vi "iscan.vi"(0 "IP adress":string="192.109.209.229", 1 "stop":bool, 2 "Channel":u8(ring)=12 items=["1", "2", "3", "4", "5", "6", "7", "8", "9", "10", "11", "12", "13", "14", "15", "16"], 3 "ISCAN Parameters":T1={"vs_initial "=TRUE, "Current_step"=0.0, "Scans"=[{" vs_initial"=FALSE, "Current_step"=0.001, "Scan_Rate"=1.0}, {" vs_initial"=FALSE, "Current_step"=-0.001, "Scan_Rate"=1.0}, {" vs_initial"=FALSE, "Current_step"=0.0, "Scan_Rate"=1.0}], "Scan_number"=2, "N_Cycles"=1, "Record_every_dI"=1e-05, "Begin_measuring_E"=0.5, "End_measuring_I"=0.75, "I_Range"=7, "E_Range"=2, "Bandwidth"=5, "em"=1, "ce"=0, "tb"=5e-05} {"tb" min=5e-05 max=1 format="%^_3e"; "ce" items=["Standard", "CE to ground"]; "End_measuring_I" min=0 max=1 format="%.2f"; "Begin_measuring_E" min=0 max=1 format="%.2f"; "Current_step" min=-150 max=150 format="%^_3e"; "N_Cycles" min=0 max=1000000; "Scan_number" min=0 max=98; "Scans"."Scan_Rate" min=0.01 max=1000 format="%^_3e"; "Scans"."Current_step" min=-150 max=150 format="%^_3e"; "E_Range" items=["±2.5V", "±5V", "±10V", "Auto"]; "Bandwidth" items=["1"=1, "2"=2, "3"=3, "4"=4, "5"=5, "6"=6, "7"=7, "8"=8, "9"=9]; "Record_every_dI" format="%^_3e"; "I_Range" items=["1pA", "1nA", "10nA", "100nA", "1µA", "10µA", "100µA", "1mA", "10mA", "100mA", "1A", "Booster"]}, 4 "Exit":bool, 5 "Start":bool, 6 "Draw":enum16{"I(Ewe)", "Ewe(t)", "I(t)"}(ring)=enum."I(t)") -> (7 "XY Graph":cluster{"Data 101":sgl[], "Data 101":sgl[]}(graph), 8 "Number of points":i32=105)   [LabVIEW 2012]
doc: "The Current scan technique (Galvanodynamic Technique) technique allows the user to perform galvanodynamic periods with different scan rates.\nIn general, in this VI, the first thing to do is to start by establishing the connection with the instrument defined by its IP adress, then load the firmware in the channel selected, get the information on the plugged channels, load protocol on a channel, start/stop the protocol, retreive data and draw the graph."
uses:
  base_xml.llb/Type Descriptor Enumeration__ogtk.ctl
panel:
  out "Device Code":i32
  out "Exit 2":bool=TRUE
  out "Data 125":sgl[][](array[numeric])=[[0.003, 0.0019739384, 6.01559e-07, 0.002076381], [0.105000004, 0.012167796, 2.1901733e-06, 0.0117511805], [0.20700002, 0.022361653, 3.975648e-06, 0.021977918], [0.30900002, 0.03255551, 5.772186e-06, 0.032090176], [0.411, 0.042749364, 7.5965745e-06, 0.042278755], [0.513, 0.052943222, 9.43279e-06, 0.052619968], [0.615, 0.06313708, 1.1011484e-05, 0.06277039], [0.717, 0.07333094, 1.3262951e-05, 0.07292081], [0.81900007, 0.08352479, 1.5135982e-05, 0.082956746], [0.92, 0.09371865, 1.6970866e-05, 0.09329796], [1.146, 0.08352479, 1.50444275e-05, 0.083796255], [1.248, 0.07333094, 1.3190472e-05, 0.07337872], [1.35, 0.06313708, 1.1359403e-05, 0.06338094], [1.4510001, 0.052943222, 9.505447e-06, 0.053039722], [1.5530001, 0.042749364, 7.704897e-06, 0.042965624], [1.6550001, 0.03255551, 5.7821057e-06, 0.03273889], [1.7570001, 0.022361653, 3.9939605e-06, 0.02243583], [1.8590001, 0.012167796, 2.2004742e-06, 0.012209094], [1.9610001, 0.0019739384, 3.9210917e-07, 0.0019060377], [2.0630002, -0.008219917, -1.42999e-06, -0.007939104], [2.1650002, -0.018413773, -3.2925293e-06, -0.01812768], [2.2670002, -0.02860763, -5.1661327e-06, -0.028087301], [2.3690002, -0.038801484, -7.0229494e-06, -0.038695633], [2.4710002, -0.048995342, -8.872135e-06, -0.048960526], [2.5730002, -0.059189197, -1.0682789e-05, -0.059149105], [2.6750002, -0.069383055, -1.2368184e-05, -0.06929952], [2.7770002, -0.07957691, -1.4145845e-05, -0.079564415], [2.8790002, -0.089770764, -1.595784e-05, -0.08963852], [2.9810002, -0.09996462, -1.7746945e-05, -0.09997973], [3.0830002, -0.11015848, -1.9597086e-05, -0.11005383], [3.1840003, -0.120352335, -2.1420525e-05, -0.1202424], [3.2860003, -0.13054618, -2.3339331e-05, -0.13024017], [3.3880002, -0.14074004, -2.5181842e-05, -0.14054324], [3.4900002, -0.1509339, -2.7039614e-05, -0.15061733], [3.5920002, -0.16112776, -2.8866867e-05, -0.16069143], [3.6940002, -0.17132162, -3.0690302e-05, -0.17118528], [3.7960002, -0.18151547, -3.246415e-05, -0.18129754], [3.8980002, -0.19170932, -3.425326e-05, -0.19167691], [4.1660004, -0.18151547, -3.2410746e-05, -0.1819081], [4.268, -0.17132162, -3.064834e-05, -0.17160504], [4.3700004, -0.16112776, -2.8840164e-05, -0.1615691], [4.472, -0.1509339, -2.6993837e-05, -0.15141869], [4.5740004, -0.14074004, -2.5170399e-05, -0.14126827], [4.676, -0.13054618, -2.3297369e-05, -0.13085073], [4.7780004, -0.120352335, -2.1454858e-05, -0.120471366], [4.88, -0.11015848, -1.9608531e-05, -0.11066438], [4.9820004, -0.09996462, -1.7731685e-05, -0.100361325], [5.084, -0.089770764, -1.5908246e-05, -0.09028722], [5.1860003, -0.07957691, -1.4138216e-05, -0.07979337], [5.288, -0.069383055, -1.23643695e-05, -0.06975743], [5.3900003, -0.059189197, -1.0510413e-05, -0.059530698], [5.491, -0.048995342, -8.728937e-06, -0.049342122], [5.5930004, -0.038801484, -6.897869e-06, -0.039191704], [5.695, -0.02860763, -5.1615543e-06, -0.029041288], [5.7970004, -0.018413773, -3.292148e-06, -0.018547434], [5.899, -0.008219917, -1.4265564e-06, -0.008549656], [6.0010004, 0.0019739384, 4.397981e-07, 0.0014481241], [6.103, 0.012167796, 2.245111e-06, 0.011636702], [6.2050004, 0.022361653, 4.0595805e-06, 0.021939758], [6.307, 0.03255551, 5.846962e-06, 0.032090176], [6.4090004, 0.042749364, 7.638159e-06, 0.04212612], [6.511, 0.052943222, 9.431646e-06, 0.05246733], [6.6130004, 0.06313708, 1.1045057e-05, 0.062579595], [6.715, 0.07333094, 1.3209546e-05, 0.07276817], [6.8170004, 0.08352479, 1.5067316e-05, 0.08303307], [6.919, 0.09371865, 1.690983e-05, 0.09318349], [7.1440005, 0.08352479, 1.5128351e-05, 0.08364362], [7.2460003, 0.07333094, 1.3301099e-05, 0.0733024], [7.3480005, 0.06313708, 1.1408995e-05, 0.06338094], [7.4490004, 0.052943222, 9.520706e-06, 0.053039726], [7.5510006, 0.042749364, 7.704897e-06, 0.042316914], [7.6530004, 0.03255551, 5.7290754e-06, 0.032624412], [7.7550006, 0.022361653, 3.9203287e-06, 0.02262663], [7.8570004, 0.012167796, 2.1073854e-06, 0.012056456], [7.9590006, 0.0019739384, 3.3221184e-07, 0.0022876323], [8.061001, -0.008219917, -1.4410538e-06, -0.007900944], [8.163, -0.018413773, -3.2478924e-06, -0.017975042], [8.265, -0.02860763, -5.089448e-06, -0.028316258], [8.367001, -0.038801484, -6.929479e-06, -0.038504835], [8.469001, -0.048995342, -8.814146e-06, -0.04869341], [8.571, -0.059189197, -1.0662569e-05, -0.059263583], [8.673, -0.069383055, -1.2417775e-05, -0.06933768], [8.775001, -0.07957691, -1.42297695e-05, -0.079144664], [8.877001, -0.089770764, -1.6053207e-05, -0.0893714], [8.979, -0.09996462, -1.7861388e-05, -0.09982709], [9.081, -0.11015848, -1.9642863e-05, -0.10990119], [9.182, -0.120352335, -2.1462487e-05, -0.12020425], [9.284, -0.13054618, -2.3247778e-05, -0.13043097], [9.386001, -0.14074004, -2.5071215e-05, -0.14046691], [9.488001, -0.1509339, -2.6944244e-05, -0.15084629], [9.59, -0.16112776, -2.8832534e-05, -0.16084407], [9.692, -0.17132162, -3.0682673e-05, -0.17129977], [9.794001, -0.18151547, -3.2525186e-05, -0.18110675], [9.896001, -0.19170932, -3.435244e-05, -0.19156244], [10.1640005, -0.18151547, -3.2357337e-05, -0.18206073], [10.266001, -0.17132162, -3.0552972e-05, -0.1716432], [10.368, -0.16112776, -2.8763869e-05, -0.16137831], [10.47, -0.1509339, -2.6936617e-05, -0.15138052], [10.5720005, -0.14074004, -2.5143696e-05, -0.14138275], [10.674001, -0.13054618, -2.3377479e-05, -0.1306981], [10.776001, -0.120352335, -2.1515893e-05, -0.12066216], [10.878, -0.11015848, -1.9719157e-05, -0.11047359], [10.9800005, -0.09996462, -1.780798e-05, -0.100513965], [11.082001, -0.089770764, -1.5946394e-05, -0.09021091], [11.184001, -0.07957691, -1.4088625e-05, -0.079869695]] format="%.2f"
  # "Instructions:\nBefore running the VI you must type a valid IP adress that corresponds to the instrument.Then press the Run button to execute this VI.\nWhile this VI is running, choose the available channel, enter the ISCAN parameters or keep the default values, then press the button start to begin the experience.\nChoose the waveform to draw (Ewe(t) or I(t) or I(Ewe) or Ec(t). You can stop the measure if you press the stop button and exit the execution if you press the exit button."
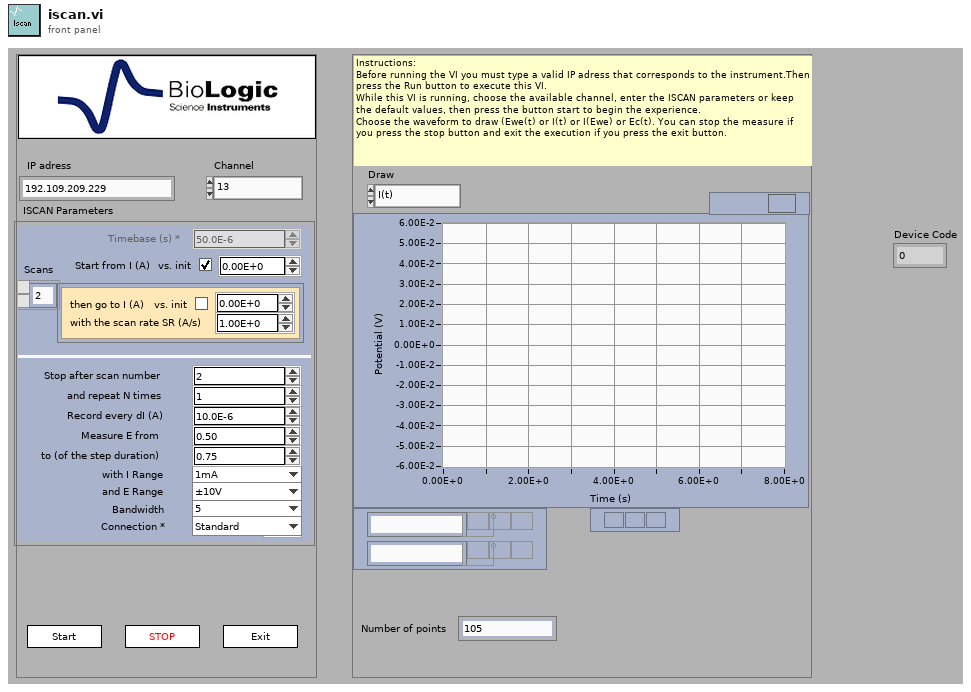
[diagram p1: front panel]
types:
  T1 = cluster{"vs_initial ":bool, "Current_step":sgl, "Scans":cluster{" vs_initial":bool, "Current_step":sgl, "Scan_Rate":sgl}[], "Scan_number":i32, "N_Cycles":i32, "Record_every_dI":sgl, "Begin_measuring_E":sgl, "End_measuring_I":sgl, "I_Range":u16, "E_Range":u16, "Bandwidth":u16, "em":u16, "ce":u16, "tb":sgl}
  T2 = typedef "Type Descriptor Enumeration__ogtk.ctl" = enum8{"<Null>", "I8", "I16", "I32", "I64", "U8", "U16", "U32", "U64", "SGL", "DBL", "EXT", "CSG", "CDB", "CXT", "0x0F", "0x10", "0x11", "0x12", "0x13", "0x14", "Enum U8", "Enum U16", "Enum U32", "Enum U64", "SGL PQ", "DBL PQ", "EXT PQ", "CSG PQ", "CDB PQ", "CXT PQ", "0x1F", "0x20", "Boolean", "0x22", "0x23", "0x24", "0x25", "0x26", "0x27", "0x28", "0x29", "0x2A", "0x2B", "0x2C", "0x2D", "0x2E", "0x2F", "String", "0x31", "Path", "Pict", "0x34", "0x35", "0x36", "DAQ", "0x38", "0x39", "0x3A", "0x3B", "0x3C", "0x3D", "0x3E", "0x3F", "Array", "0x41", "0x42", "0x43", "0x44", "0x45", "0x46", "0x47", "0x48", "0x49", "0x4A", "0x4B", "0x4C", "0x4D", "0x4E", "0x4F", "Cluster", "0x51", "0x52", "Variant", "Waveform", "0x55", "0x56", "0x57", "0x58", "0x59", "0x5A", "0x5B", "0x5C", "0x5D", "0x5E", "0x5F", "0x60", "0x61", "0x62", "0x63", "0x64", "0x65", "0x66", "0x67", "0x68", "0x69", "0x6A", "0x6B", "0x6C", "0x6D", "0x6E", "0x6F", "Refnum"}
  T3 = cluster{"Data Type":T2, "Format String":string}[]
  T4 = cluster{"Channel":i32, "BoardVersion":i32, "BoardSerialCode":i32, "FirmwareCode":i32, "FirmwareVersion":i32, "XilinxVersion":i32, "AmpCode":i32, "NbAmp":i32, "LcBoard":i32, "Zboard":i32, "MuxBoard":i32, "GPRAboard":i32, "MemSize":i32, "MemFilled":i32, "state":i32, "MaxIRange":i32, "MinIRange":i32, "MaxBandwidth":i32, "NbOfTechniques":i32}
  T5 = cluster{" vs_initial":bool, "Current_step":sgl, "Scan_Rate":sgl}[]
  T6 = cluster{" vs_initial":bool, "Current_step":sgl, "Scan_Rate":sgl}
  T7 = cluster{"Label":string, "type":i32, "valeur":u32, "index":i32}[]
  T8 = cluster{"IRQskipped":i32, "NbRaws":i32, "NbCols":i32, "Technique Index":i32, "TechniqueID":i32, "PrcessIndex":i32, "loop":i32, "StartTime":dbl, "MuxPad":i32}
  T9 = cluster{"State":i32, "MemFilled":i32, "TimeBase":sgl, " Ewe":sgl, " EweRangeMin":sgl, " EweRangeMax":sgl, "Ece":sgl, "EceRangeMin":sgl, "EceRangeMax":sgl, "Eoverflow":i32, "I":sgl, "IRange":i32, "Ioverflow":i32, "ElapsedTime":sgl, "Freq":sgl, "Rcomp":sgl, "Saturation":sgl, "OptErr":i32, "OptPos":i32}
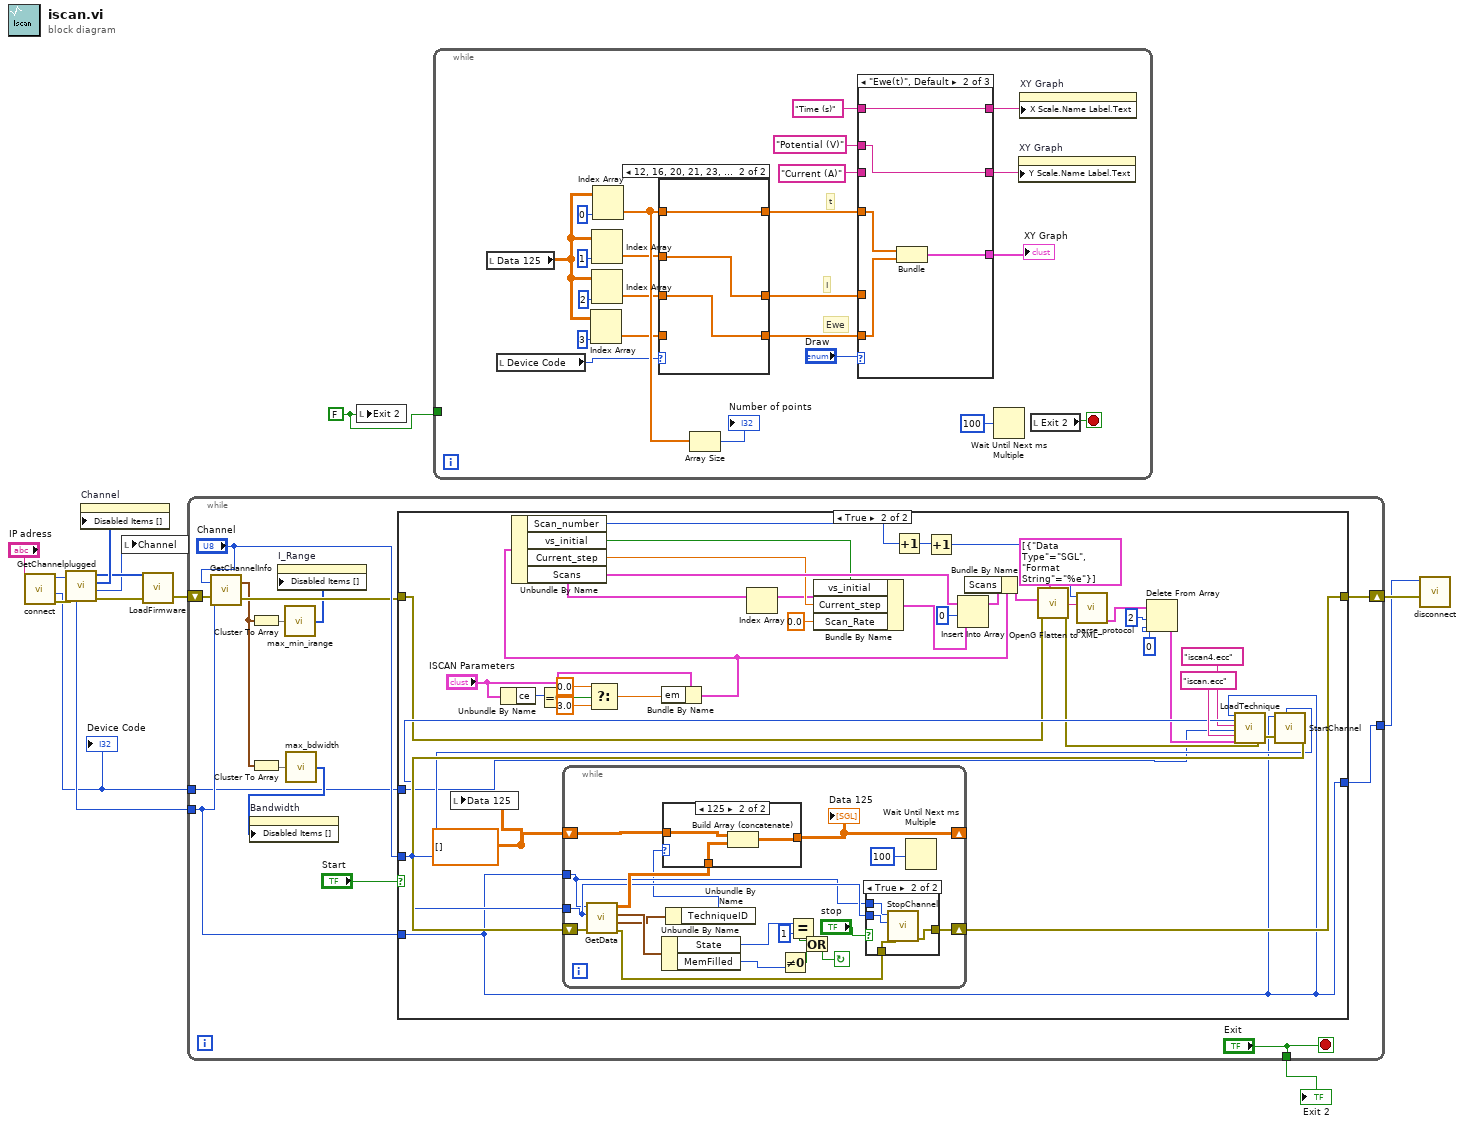
[diagram p0: block diagram]
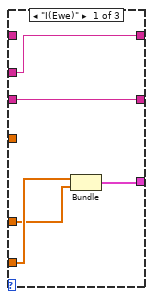
[diagram p3: hidden frame]
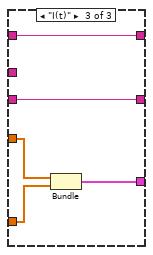
[diagram p4: hidden frame]
diagram:
  w12 = FALSE ("Exit 2")
  n1 = call "connect.vi"("IP"="IP adress") -> ("error out"=w10:errorcluster, "Device Code"=w1:i32, "ID"=w3:i32)  [unwired: 7 in, 1 out]
  "Device Code" <- w1
  n2 = call "GetChannelplugged.vi"("error in (no error)"=w10, "ID"=w3) -> ("error out"=w7:errorcluster, "First channel"=w5:i32, "Disabled channels"=w9:i32[], "Plugged channels"=w8:i32[])  [unwired: 6 in]
  n3 = property on="Channel" class="Ring (strict)"("Disabled Items []"=w9) -> ()  [unwired: 2 in, 2 out]
  n4 = local write "Channel"(w5) -> ()
  n5 = call "LoadFirmware.vi"("error in (no error)"=w7, "Channels"=w8, "ID"=w3) -> ("error out"=w4:errorcluster)  [unwired: 7 in, 1 out]
  n6 = while {
    shift-right: [w26] -> w11
    shift-left: w4 -> [w23]
    tunnel: ["Exit"] -> w13
    tunnel: w3 -> [w16]
    tunnel: [w15] -> w2
    tunnel: w1 -> [w14]
    stop <- "Exit" stop-if-true
    n7 = call "GetChannelInfo.vi"("error in (no error)"=w23, "Channel"="Channel", "ID"=w16) -> ("error out"=w22:errorcluster, "Channel information"=w19:T4)  [unwired: 7 in]
    n8 = Cluster To Array(cluster=w19) -> (array=w21:i32[])
    n9 = Cluster To Array(cluster=w19) -> (array=w20:i32[])
    n10 = call "max_min_irange.vi"("resources"=w21) -> ("disabled ranges"=w17:i32[])
    n11 = property on="I_Range" class="Ring (strict)"("Disabled Items []"=w17) -> ()  [unwired: 2 in, 2 out]
    n12 = call "max_bdwidth.vi"("resources"=w20) -> ("disabled ranges"=w18:i32[])
    n13 = property on="Bandwidth" class="Ring (strict)"("Disabled Items []"=w18) -> ()  [unwired: 2 in, 2 out]
    n14 = case shown="True" "Start" {
      tunnel: "Channel" -> [_ w60]
      tunnel: [w29 w62] -> w26
      tunnel: w22 -> [w29 w57]
      tunnel: w16 -> [w28 w42]
      tunnel: [w28 w42] -> w15
      tunnel: w14 -> [_ w38]
      frame False {
      }
      frame True {
        w61 = sgl[][] []
        n15 = local write "Data 125"(w61) -> ()
        n16 = Unbundle By Name("ISCAN Parameters") -> ("ce"=w33:u16)
        n17 = Equal To 0?(x=w33) -> (x = 0?=w32:bool)
        n18 = Select(t=0.0, s=w32, f=3.0) -> (s? t:f=w36:dbl)
        n19 = Bundle By Name(cluster="ISCAN Parameters", "em"=w36) -> (w30:T1)
        n20 = Unbundle By Name(w30) -> ("Scan_number"=w40:i32, "vs_initial"=w46:bool, "Current_step"=w47:sgl, "Scans"=w50:T5)
        n21 = Index Array(array=w50) -> (element=w44:T6)  [unwired: 1 in]
        n22 = Bundle By Name(cluster=w44, "vs_initial"=w46, "Current_step"=w47, "Scan_Rate"=sgl 0.0) -> (w48:T6)
        n23 = Increment(x=w40) -> (x+1=w41:i32)
        n24 = Increment(x=w41) -> (x+1=w39:i32)
        n25 = Insert Into Array(array=w50, index=0 ("indice"), new element=w48) -> (w51:T5)
        n26 = Bundle By Name(cluster=w30, "Scans"=w51) -> (w43:T1)
        n27 = call "OpenG Flatten to XML.vi"("Type Formats (default)"=T3 [{"Data Type"=enum."SGL", "Format String"="%e"}] ("Type Formats"), "error in (no error)"=w57, "LabVIEW Data"=w43) -> ("error out"=w56:errorcluster, "XML String"=w58:string)  [unwired: 7 in]
        n28 = call "parse_protocol.vi"("XML String In"=w58, "index array"=w39) -> ("Params Values"=w53:T7)  [unwired: 7 in]
        n29 = Delete From Array(array=w53, length=2 ("longueur"), index=0 ("indice")) -> (array with subset deleted=w52:T7)  [unwired: 1 out]
        n30 = call "LoadTechnique.vi"("ID"=w42, "Selected Channel"=w60, "FName4"="iscan4.ecc" ("FName"), "Device Code"=w38, "FName"="iscan.ecc", "Protocol Parameters"=w52, "error in (no error)"=w56) -> ("error out"=w64:errorcluster)  [unwired: 12 in]
        n31 = call "StartChannel.vi"("error in (no error)"=w64, "Channel"=w60, "ID"=w42) -> ("error out"=w63:errorcluster)  [unwired: 8 in]
        n32 = while {
          shift-right: [w78] -> w62
          shift-left: w63 -> [w81]
          shift-right: [w75] -> _
          shift-left: w61 -> [w76]
          tunnel: w60 -> [w72]
          tunnel: w42 -> [w71]
          stop <- w79 continue-if-true
          n33 = call "GetData.vi"("error in (no error)"=w81, "Channel"=w72, "ID"=w71) -> ("error out"=w74:errorcluster, "Data information"=w66:T8, "Current values"=w67:T9, "Data"=w77:dbl[][])  [unwired: 5 in]
          n34 = Unbundle By Name(w67) -> ("State"=w68:i32, "MemFilled"=w69:i32)
          n35 = Unbundle By Name(w66) -> ("TechniqueID"=w70:i32)
          n36 = case shown="125" w70 {
            tunnel: w77 -> [_ w93]
            tunnel: w76 -> [w90 w92]
            tunnel: [w90 w91] -> w75
            frame 0, Default {
            }
            frame 125 {
              n37 = Build Array (concatenate)(w92, w93) -> (w91:dbl[][])
            }
          }
          "Data 125" <- w75
          n38 = Not Equal To 0?(x=w69) -> (x != 0?=w82:bool)
          n39 = Equal?(x=w68, y=1) -> (x = y?=w83:bool)
          n40 = Or(x=w83, y=w82) -> (x .or. y?=w79:bool)
          n41 = case shown="True" "stop" {
            tunnel: [w85 w89] -> w78
            tunnel: w74 -> [w85 w88]
            tunnel: w72 -> [_ w87]
            tunnel: w71 -> [_ w86]
            frame False {
            }
            frame True {
              n42 = call "StopChannel.vi"("error in (no error)"=w88, "Channel"=w87, "ID"=w86) -> ("error out"=w89:errorcluster)  [unwired: 8 in]
            }
          }
          n43 = Wait Until Next ms Multiple(millisecond multiple=u32 100) -> ()  [unwired: 1 out]
        }
      }
    }
  }
  "Exit 2" <- w13
  n44 = local write "Exit 2"(w12) -> ()
  n45 = while {
    tunnel: w12 -> [_]
    stop <- w115 stop-if-true
    # "Ewe"
    # "I"
    # "t"
    n46 = local read "Data 125"() -> (w103:sgl[][])
    n47 = local read "Device Code"() -> (w94:i32)
    n48 = Index Array(array=w103, index (col)=3 ("Index")) -> (element=w96:sgl[])  [unwired: 1 in]
    n49 = Index Array(array=w103, index (col)=1 ("Index")) -> (element=w99:sgl[])  [unwired: 1 in]
    n50 = Index Array(array=w103, index (col)=2 ("Index")) -> (element=w98:sgl[])  [unwired: 1 in]
    n51 = Index Array(array=w103, index (col)=0 ("Index")) -> (element=w101:sgl[])  [unwired: 1 in]
    n52 = case shown="12, 16, 20, 21, 23, 27" w94 {
      tunnel: w101 -> [w119 w122]
      tunnel: [w119 w122] -> w100
      tunnel: w99 -> [_ w121]
      tunnel: w98 -> [w118 w120]
      tunnel: [w118 w121] -> w97
      tunnel: w96 -> [w117 _]
      tunnel: [w117 w120] -> w95
      frame 0, Default {
      }
      frame 12, 16, 20, 21, 23, 27 {
      }
    }
    n53 = Array Size(array=w101) -> (size(s)=→"Number of points":i32)
    n54 = case shown="\"Ewe(t)\", Default" "Draw" {
      tunnel: w100 -> [_ w132 w137]
      tunnel: w97 -> [w124 _ w136]
      tunnel: [w123 w128 w133] -> w102
      tunnel: "Potential (V)" ("Y Scale.Name Label.Text") -> [w127 w131 _]
      tunnel: "Current (A)" ("Y Scale.Name Label.Text") -> [w126 _ w135]
      tunnel: [w126 w131 w135] -> w107
      tunnel: [w127 w130 w134] -> w106
      tunnel: "Time (s)" ("Y Scale.Name Label.Text") -> [_ w130 w134]
      tunnel: w95 -> [w125 w129 _]
      frame "I(Ewe)" {
        n55 = Bundle("Data 125"=w125, "Data 125"=w124) -> (w123:cluster{"Data 125":sgl[], "Data 125":sgl[]})  [unwired: 1 in]
      }
      frame "Ewe(t)", Default {
        n56 = Bundle("Data 125"=w132, "Data 125"=w129) -> (w128:cluster{"Data 125":sgl[], "Data 125":sgl[]})  [unwired: 1 in]
      }
      frame "I(t)" {
        n57 = Bundle("Data 125"=w137, "Data 125"=w136) -> (w133:cluster{"Data 125":sgl[], "Data 125":sgl[]})  [unwired: 1 in]
      }
    }
    "XY Graph" <- w102
    n58 = Wait Until Next ms Multiple(millisecond multiple=u32 100) -> ()  [unwired: 1 out]
    n59 = property on="XY Graph" class="XYGraph (strict)"("Y Scale.Name Label.Text"=w107) -> ()  [unwired: 2 in, 2 out]
    n60 = property on="XY Graph" class="XYGraph (strict)"("X Scale.Name Label.Text"=w106) -> ()  [unwired: 2 in, 2 out]
    n61 = local read "Exit 2"() -> (w115:bool)
  }
  n62 = call "disconnect.vi"("error in (no error)"=w11, "ID"=w2) -> ()  [unwired: 9 in, 1 out]
